vi "Intensity Graph Linecut (Vertical).vi"(8 "error in (no error)":errorcluster, 9 "width (vertical)":dbl, 11 "graph_utilities in":refnum<class "graph_utilities.lvclass">) -> (0 "error out":errorcluster, 3 "graph_utilities out":refnum<class "graph_utilities.lvclass">)   [LabVIEW 2016, in "graph_utilities.lvclass"]
uses:
  graph_utilities.lvclass
  <vilib>/Analysis/baseanly.llb/A x Vector.vi
  <vilib>/Analysis/NI_AALBase.lvlib
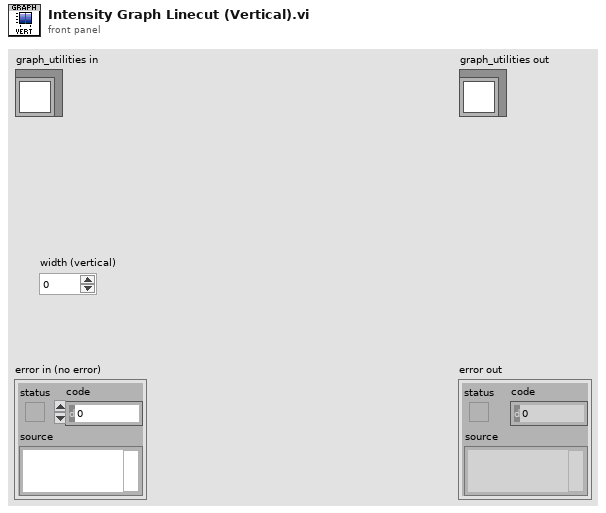
[diagram p1: front panel]
types:
  T1 = typedef "LVPointDoubleTypeDef.ctl" = cluster{"X":dbl, "Y":dbl}
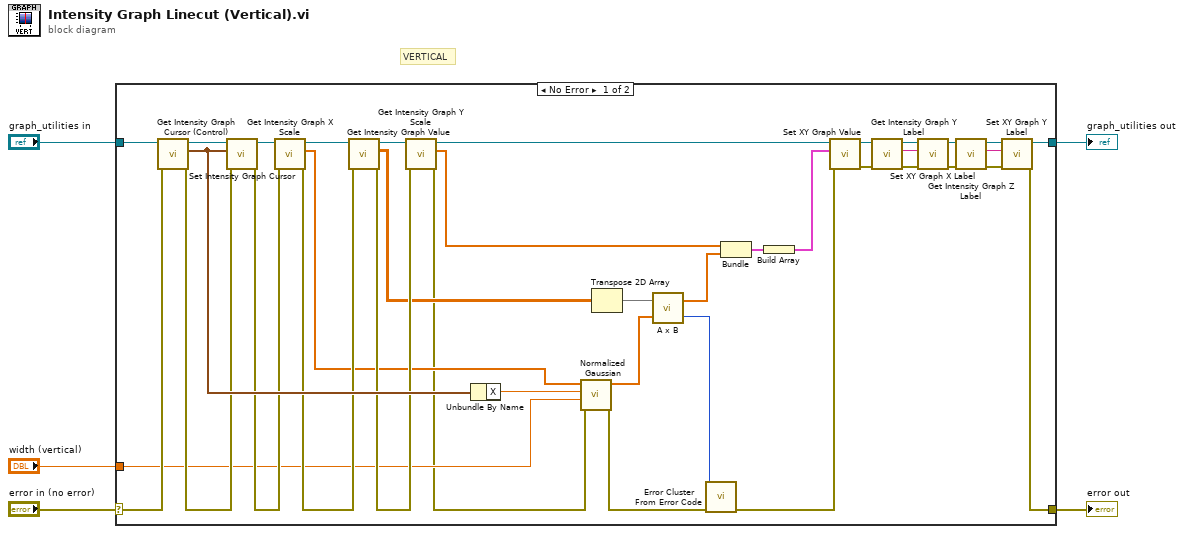
[diagram p0: block diagram]
diagram:
  # "VERTICAL"
  n1 = case shown="No Error" "error in (no error)" {
    selector: "error in (no error)" -> [w36 w45]
    tunnel: [w7 w45] -> w4
    tunnel: [w6 w44] -> w2
    tunnel: "graph_utilities in" -> [w39 w44]
    tunnel: "width (vertical)" -> [w25 _]
    frame No Error {
      n2 = call "Get Intensity Graph Cursor (Control).vi"("error in (no error)"=w36, "graph_utilities in"=w39) -> ("error out"=w35:errorcluster, "Cursor.Cursor Position"=w37:T1, "graph_utilities out"=w40:refnum<class "graph_utilities.lvclass">)  [unwired: 7 in]
      n3 = call "Set Intensity Graph Cursor.vi"("error in (no error)"=w35, "Cursor.Cursor Position"=w37, "graph_utilities in"=w40) -> ("error out"=w34:errorcluster, "graph_utilities out"=w38:refnum<class "graph_utilities.lvclass">)  [unwired: 7 in]
      n4 = call "Get Intensity Graph X Scale.vi"("error in (no error)"=w34, "graph_utilities in"=w38) -> ("error out"=w31:errorcluster, "X Scale"=w27:dbl[], "graph_utilities out"=w33:refnum<class "graph_utilities.lvclass">)  [unwired: 6 in, 1 out]
      n5 = call "Get Intensity Graph Value.vi"("error in (no error)"=w31, "graph_utilities in"=w33) -> ("error out"=w30:errorcluster, "Value"=w29:dbl[][], "graph_utilities out"=w32:refnum<class "graph_utilities.lvclass">)  [unwired: 7 in]
      n6 = call "Get Intensity Graph Y Scale.vi"("error in (no error)"=w30, "graph_utilities in"=w32) -> ("error out"=w23:errorcluster, "Y Scale"=w28:dbl[], "graph_utilities out"=w20:refnum<class "graph_utilities.lvclass">)  [unwired: 6 in, 1 out]
      n7 = Unbundle By Name(w37) -> ("X"=w26:dbl)
      n8 = call "Normalized Gaussian.vi"("error in (no error)"=w23, "width (c)"=w25, "position (b)"=w26, "Scale"=w27) -> ("error out"=w22:errorcluster, "Normalized Gaussian"=w24:dbl[])  [unwired: 6 in]
      n9 = Transpose 2D Array(2D array=w29) -> (transposed array=w43:dbl[][])
      n10 = call-poly <vilib>:"A x B.vi"("Vector"=w24, "A"=w43) -> ("error"=w41:i32, "A x Vector"=w42:dbl[])
      n11 = call <vilib>:"Error Cluster From Error Code.vi"("error in (no error)"=w22, "error code (0)"=w41) -> ("error out"=w19:errorcluster)  [unwired: 7 in]
      n12 = Bundle("Y Scale"=w28, "A x Vector"=w42) -> (w21:cluster{"Y Scale":dbl[], "A x Vector":dbl[]})  [unwired: 1 in]
      n13 = Build Array(w21) -> (w18:cluster{"Y Scale":dbl[], "A x Vector":dbl[]}[])
      n14 = call "Set XY Graph Value.vi"("error in (no error)"=w19, "Value"=w18, "graph_utilities in"=w20) -> ("error out"=w8:errorcluster, "graph_utilities out"=w13:refnum<class "graph_utilities.lvclass">)  [unwired: 7 in]
      n15 = call "Get Intensity Graph Y Label.vi"("error in (no error)"=w8, "graph_utilities in"=w13) -> ("error out"=w11:errorcluster, "Y Label"=w14:string, "graph_utilities out"=w12:refnum<class "graph_utilities.lvclass">)  [unwired: 7 in]
      n16 = call "Set XY Graph X Label.vi"("error in (no error)"=w11, "X Label"=w14, "graph_utilities in"=w12) -> ("error out"=w9:errorcluster, "graph_utilities out"=w10:refnum<class "graph_utilities.lvclass">)  [unwired: 7 in]
      n17 = call "Get Intensity Graph Z Label.vi"("error in (no error)"=w9, "graph_utilities in"=w10) -> ("error out"=w15:errorcluster, "Z Label"=w17:string, "graph_utilities out"=w16:refnum<class "graph_utilities.lvclass">)  [unwired: 7 in]
      n18 = call "Set XY Graph Y Label.vi"("error in (no error)"=w15, "Y Label"=w17, "graph_utilities in"=w16) -> ("error out"=w7:errorcluster, "graph_utilities out"=w6:refnum<class "graph_utilities.lvclass">)  [unwired: 7 in]
    }
    frame Error {
    }
  }
  "error out" <- w4
  "graph_utilities out" <- w2
